vi "instance count allowed.vi"(8 "error in":errorcluster, 11 "Custom Controller Module configuration in":refnum<class "Custom Controller Module configuration.lvclass">) -> (0 "error out":errorcluster, 2 "instances allowed":i32, 3 "Custom Controller Module configuration out":refnum<class "Custom Controller Module configuration.lvclass">)   [LabVIEW 2013, in "Custom Controller Module configuration.lvclass"]
uses:
  Custom Controller Module configuration.lvclass
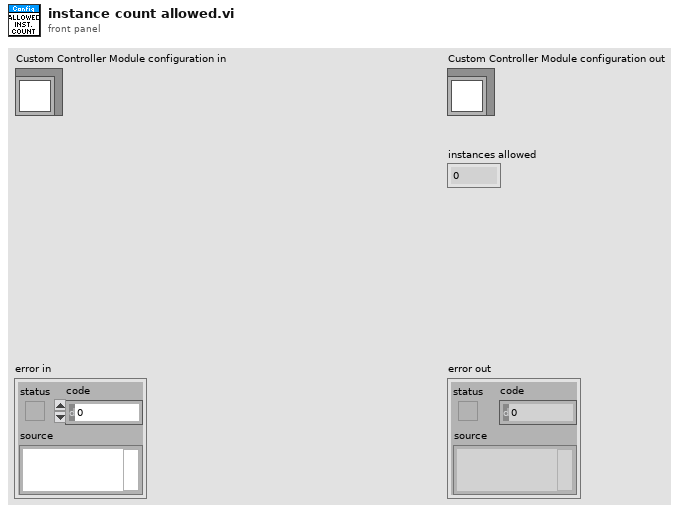
[diagram p1: front panel]
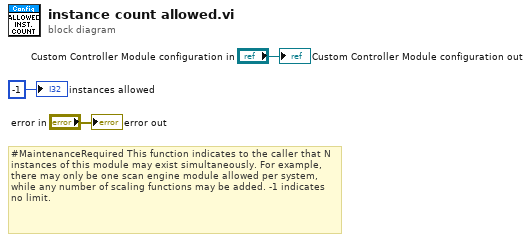
[diagram p0: block diagram]
diagram:
  # "#MaintenanceRequired This function indicates to the caller that N instances of this module may exist simultaneously. For example, there may only be one scan engine module allowed per system, while any number of scaling functions may be added. -1 indicates no limit."
  "error out" <- "error in"
  "Custom Controller Module configuration out" <- "Custom Controller Module configuration in"
  "instances allowed" <- -1 ("instances allowed")
